vi "Motor Button Setpoint.vi"(0 "Speed":dbl, 8 "Subtract":bool, 9 "ADD":bool) -> ()   [LabVIEW 2014]
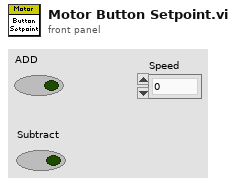
[diagram p1: front panel]
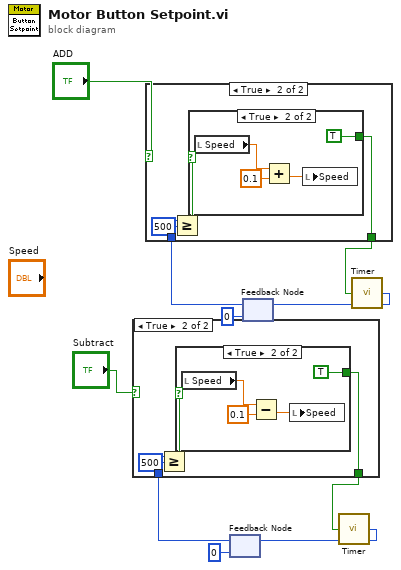
[diagram p0: block diagram]
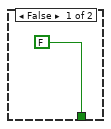
[diagram p2: hidden frame]
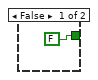
[diagram p3: hidden frame]
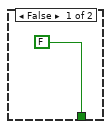
[diagram p4: hidden frame]
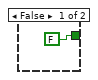
[diagram p5: hidden frame]
diagram:
  n1 = feedback #1(u64 0 ("Time elapsed")) -> (w8:u64)
  n2 = case shown="True" "Subtract" {
    tunnel: [FALSE w15] -> w6
    tunnel: w8 -> [_ w14]
    frame False {
    }
    frame True {
      n3 = Greater Or Equal?(x=w14, y=u64 500) -> (x >= y?=w12:bool)
      n4 = case shown="True" w12 {
        tunnel: [FALSE TRUE] -> w15
        frame False {
        }
        frame True {
          n5 = local read "Speed"() -> (w20:dbl)
          n6 = Subtract(x=w20, y=0.1) -> (x-y=w19:dbl)
          n7 = local write "Speed"(w19) -> ()
        }
      }
    }
  }
  n8 = feedback #2(u64 0 ("Time elapsed")) -> (w4:u64)
  n9 = case shown="True" "ADD" {
    tunnel: [FALSE w25] -> w2
    tunnel: w4 -> [_ w24]
    frame False {
    }
    frame True {
      n10 = Greater Or Equal?(x=w24, y=u64 500) -> (x >= y?=w22:bool)
      n11 = case shown="True" w22 {
        tunnel: [FALSE TRUE] -> w25
        frame False {
        }
        frame True {
          n12 = local read "Speed"() -> (w30:dbl)
          n13 = Add(x=w30, y=0.1) -> (x+y=w28:dbl)
          n14 = local write "Speed"(w28) -> ()
        }
      }
    }
  }
  n15 = call "Timer.vi"("Set Timer"=w6) -> ("Time elapsed"=w7:u64)
  n16 = feedback-in #1(w7) -> ()
  n17 = call "Timer.vi"("Set Timer"=w2) -> ("Time elapsed"=w3:u64)
  n18 = feedback-in #2(w3) -> ()
